vi "Single Unpress.vi"(11 "Button In":bool) -> (3 "Button out":bool)   [LabVIEW 2015]
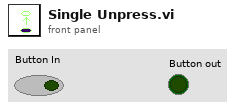
[diagram p1: front panel]
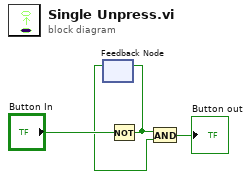
[diagram p0: block diagram]
diagram:
  n1 = feedback #1() -> (w2:bool)  [unwired: 1 in]
  n2 = Not(x="Button In") -> (.not. x?=w1:bool)
  n3 = feedback-in #1(w1) -> ()
  n4 = And(x=w1, y=w2) -> (x .and. y?=→"Button out":bool)
